vi "R&S RF Off.vi"(4 "error in (no error)":errorcluster, 7 "address":string) -> (0 "error out":errorcluster, 3 "address out":string)   [LabVIEW 2019]
doc: "This device configures the Rohde & Schwarz RF Generator for use. The central frequency, modulation, RF power, and GPIB address are taken from the QCA Global."
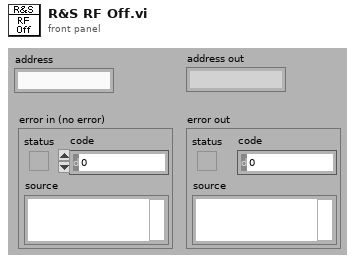
[diagram p1: front panel]
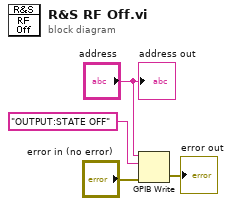
[diagram p0: block diagram]
diagram:
  n1 = GPIB Write(0:"address", 1:"OUTPUT:STATE OFF", 3:"error in (no error)") -> (6:→"error out":errorcluster)  [unwired: 2 in, 1 out]
  "address out" <- "address"
